vi "opcode response to string.vi"(11 "Data Received":u8[](array[numeric])) -> (3 "Response String":string)   [LabVIEW 2020]
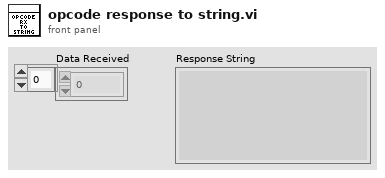
[diagram p1: front panel]
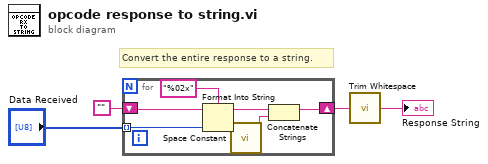
[diagram p0: block diagram]
diagram:
  # "Convert the entire response to a string."
  n1 = for {
    shift-right: [w6] -> w2
    shift-left: "" -> [w10]
    tunnel: "Data Received" -> [w5] mode=indexing
    n2 = Format Into String(format string="%02x", initial string=w10, w5) -> (resulting string=w8:string)  [unwired: 1 in, 1 out]
    n3 = call <vilib>:"Space Constant.vi"() -> ("String"=w7:string)
    n4 = Concatenate Strings(w8, w7) -> (w6:string)
  }
  n5 = call <vilib>:"Trim Whitespace.vi"("string"=w2) -> ("trimmed string"=→"Response String":string)  [unwired: 1 in]
